vi "sendMessage.vi"(8 "error in (no error)":errorcluster, 9 "data":variant, 10 "message":string, 11 "BoolNotifierTaskChannel in":refnum<class "BoolNotifierTaskChannel.lvclass">) -> (0 "error out":errorcluster, 3 "BoolNotifierTaskChannel out":refnum<class "BoolNotifierTaskChannel.lvclass">)   [LabVIEW 2023, in "TLC_Daemon.lvlib" / "BoolNotifierTaskChannel.lvclass"]
uses:
  BoolNotifierTaskChannel.lvclass
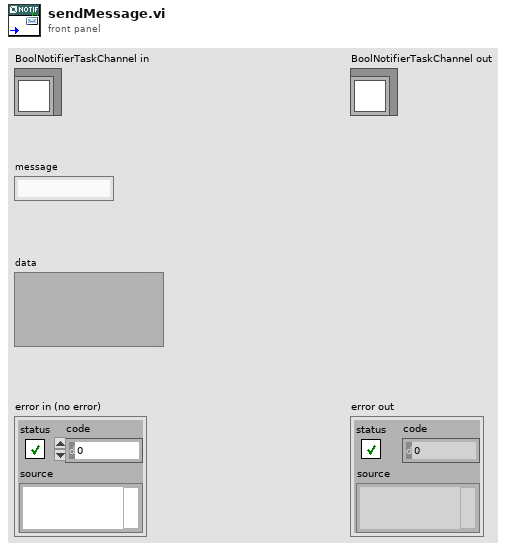
[diagram p1: front panel]
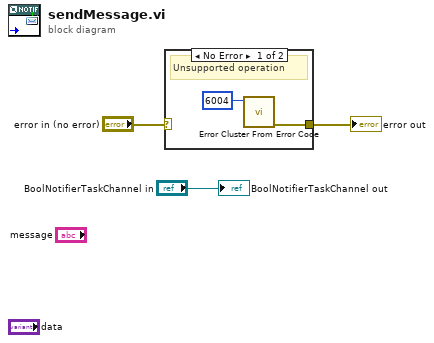
[diagram p0: block diagram]
diagram:
  n1 = case shown="No Error" "error in (no error)" {
    selector: "error in (no error)" -> [_ w6]
    tunnel: [w4 w6] -> w1
    frame No Error {
      # "Unsupported operation"
      n2 = call <vilib>:"Error Cluster From Error Code.vi"("error code (0)"=6004) -> ("error out"=w4:errorcluster)  [unwired: 8 in]
    }
    frame Error {
    }
  }
  "error out" <- w1
  "BoolNotifierTaskChannel out" <- "BoolNotifierTaskChannel in"
